vi "Tetra_CalAdc.vi"(0 "COMPORT":refnum<visa-resource-name>="COM4", 5 "error in (no error)":errorcluster, 9 "ADC_Cal_Function":i32(ring) items=["CalADC", "ReadADC"], 11 "Open Ser(t)":bool, 13 "Close Ser(t)":bool) -> (10 "Success":bool, 12 "read":string="caladc -s\r\nfinal caladc delay: 0x0000CCB9* mag: 2 2 2 2\r\n>\r\n", 14 "comport":refnum<visa-resource-name>="COM4", 16 "cal_adc_mag":string="mag: 2 2 2 2", 17 "cal_adc_delay":string="caladc delay: 0x0000CCB9* ", 19 "error out":errorcluster)   [LabVIEW 2018]
doc: "This example performs writes and reads on a serial port, as directed by the user. You can press the Write and Read buttons, and change the Read Count, while the example is running.\n\nThe parameters set for the serial port must match the parameters of the connected instrument or device. In this example, the Read Count parameter specifies the number of bytes that the serial port reads. If there were more bytes at the port than the specified number, those bytes would not be read. If there were less bytes at the port than the specified number, you would receive a timeout error.\n\nThis example expands upon the flow control options for XON and XOFF, allowing the user to choose those control characters. Also, the user can enable or disable a termination character. Some devices require a termination character in order to identify the end of command strings. Some devices send a termination character to signify the end of data to be read. This example shows how you can end the Read operation once a termination character is detected in the buffer and/or append a termination character at the end of the Write data."
uses:
  <vilib>/Utility/error.llb/whitespace.ctl
panel:
  out "x-y":dbl=12.528091899992432
  out "cmd":string="caladc -s"
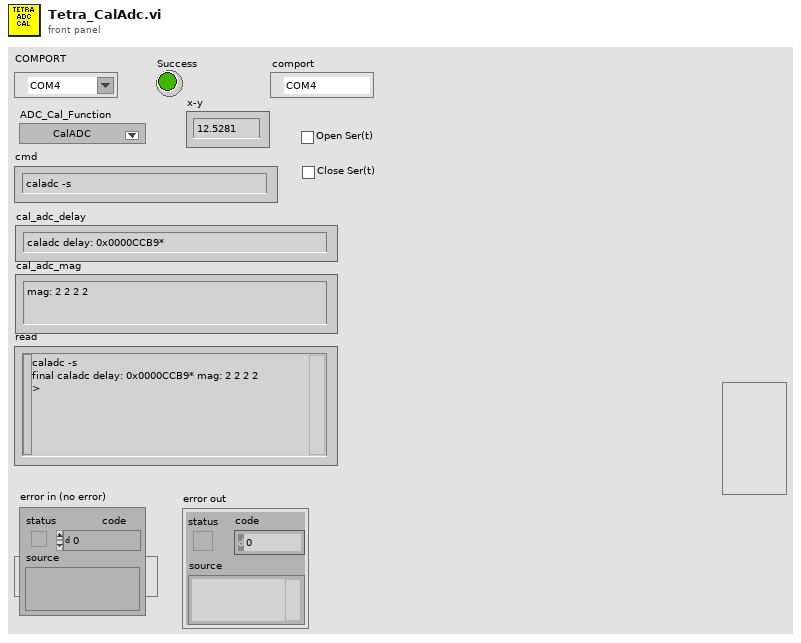
[diagram p1: front panel]
types:
  T1 = typedef "whitespace.ctl" = u16
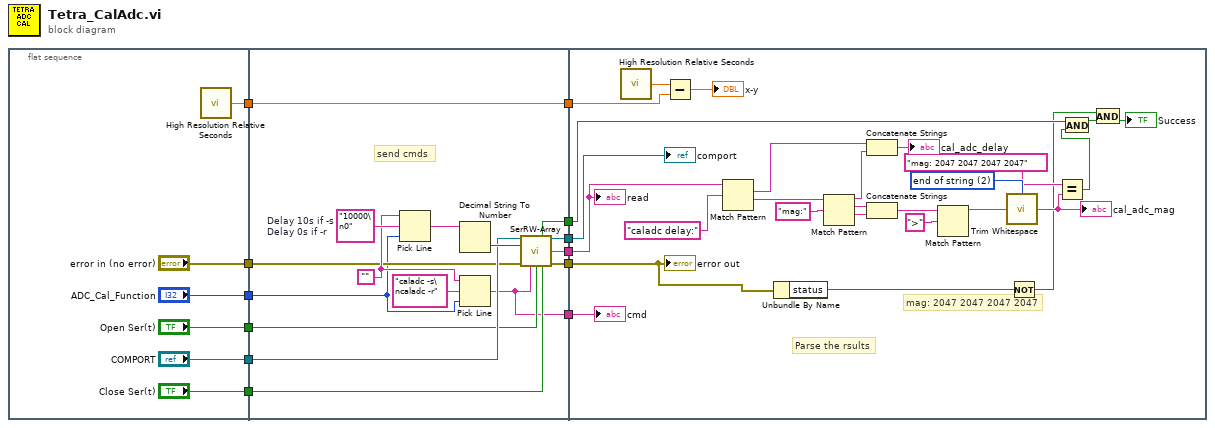
[diagram p0: block diagram]
diagram:
  n1 = flat-sequence {
    tunnel: ["COMPORT"] -> w12
    tunnel: ["Close Ser(t)"] -> w11
    tunnel: ["Open Ser(t)"] -> w10
    tunnel: ["error in (no error)"] -> w9
    tunnel: ["ADC_Cal_Function"] -> w7
    tunnel: [w13] -> w2
    tunnel: w12 -> [w29]
    tunnel: w11 -> [w28]
    tunnel: w10 -> [w27]
    tunnel: w9 -> [w26]
    tunnel: [w25] -> w8
    tunnel: w7 -> [w24]
    tunnel: [w23] -> w6
    tunnel: [w22] -> w5
    tunnel: [w21] -> w4
    tunnel: [w20] -> w3
    tunnel: w2 -> [w19]
    tunnel: [w19] -> w1
    tunnel: w8 -> [w53]
    tunnel: w6 -> [w52]
    tunnel: w5 -> [w51]
    tunnel: w4 -> [w50]
    tunnel: w3 -> [w37]
    tunnel: w1 -> [w44]
    frame #0 {
      n2 = call <vilib>:"High Resolution Relative Seconds.vi"() -> ("relative seconds"=w13:dbl)
    }
    frame #1 {
      w32 = "10000\n0"  # Delay 10s if -s Delay 0s if -r
      w31 = ""
      # "send cmds"
      n3 = Pick Line(string ("")=w31, multi-line string=w32, line index=w24) -> (output string=w33:string)
      n4 = Decimal String To Number(string=w33) -> (number=w34:i32)  [unwired: 2 in, 1 out]
      n5 = Pick Line(string ("")=w31, multi-line string="caladc -s\ncaladc -r", line index=w24) -> (output string=w23:string)
      n6 = call "SerRW-Array.vi"("COMPORT"=w29, "Delay Time (ms)"=w34, "error in (no error)"=w26, "Command ( ; seperation)"=w23, "Open Serial"=w27, "Close Serial"=w28) -> ("All Success"=w22:bool, "comport"=w25:refnum<visa-resource-name>, "string"=w21:string, "error out"=w20:errorcluster)  [unwired: 4 in, 2 out]
    }
    frame #2 {
      w46 = T1 2 items=["both", "start of string", "end of string"] ("location (both)")
      # "mag: 2047 2047 2047 2047"
      # "Parse the rsults"
      n7 = call <vilib>:"High Resolution Relative Seconds.vi"() -> ("relative seconds"=w45:dbl)
      n8 = Subtract(x=w45, y=w44) -> (x-y=→"x-y":dbl)
      n9 = Match Pattern(string=w50, regular expression="caladc delay:") -> (match substring=w59:string, after substring=w56:string)  [unwired: 1 in, 2 out]
      n10 = Unbundle By Name(w37) -> ("status"=w36:bool)
      n11 = Match Pattern(string=w56, regular expression="mag:") -> (before substring=w57:string, match substring=w60:string, after substring=w61:string)  [unwired: 1 in, 1 out]
      n12 = Concatenate Strings(w59, w57) -> (→"cal_adc_delay":string)
      n13 = Concatenate Strings(w60, w61) -> (w48:string)
      n14 = Match Pattern(string=w48, regular expression=">") -> (before substring=w47:string)  [unwired: 1 in, 3 out]
      n15 = call <vilib>:"Trim Whitespace.vi"("string"=w47, "location (both)"=w46) -> ("trimmed string"=w42:string)
      "cal_adc_mag" <- w42
      n16 = Not(x=w36) -> (.not. x?=w35:bool)
      n17 = Equal?(x="mag: 2047 2047 2047 2047", y=w42) -> (x = y?=w39:bool)
      n18 = And(x=w51, y=w39) -> (x .and. y?=w40:bool)
      n19 = And(x=w35, y=w40) -> (x .and. y?=→"Success":bool)
      "read" <- w50
      "comport" <- w53
      "error out" <- w37
      "cmd" <- w52
    }
  }
